vi "OCT_Run_sub.vi"(11 "saveing method":string(combo)="SaveQueueImages") -> (3 "Lumedica report":string)   [LabVIEW 2021]
uses:
  <vilib>/Instr/_visa.llb/Select Event Type.ctl
  <vilib>/Instr/_visa.llb/VISA Configure Serial Port (Instr).vi
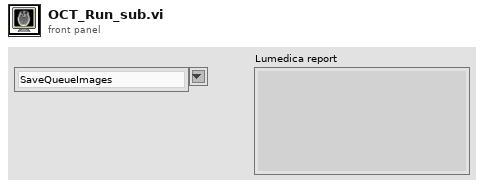
[diagram p1: front panel]
types:
  T1 = typedef "Select Event Type.ctl" = u32
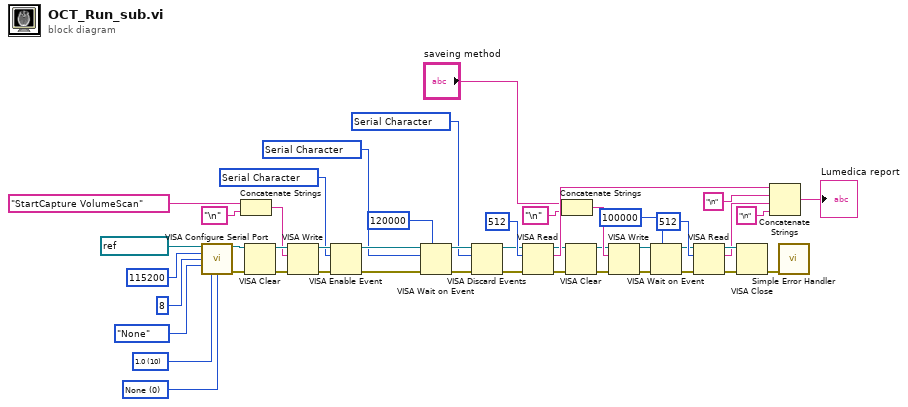
[diagram p0: block diagram]
diagram:
  w6 = T1 1073684533 items=["Service Request"=1073684491, "Trigger"=3221168138, "Clear"=1073684493, "VXI Signal"=1073684512, "VXI/VME Interrupt"=3221168161, "VXI/VME Sysfail"=1073684509, "VXI/VME Sysreset"=1073684510, "GPIB CIC"=1073684498, "GPIB Talk"=1073684499, "GPIB Listen"=1073684500, "PXI Interrupt"=1073684514, "Serial Break"=1073684515, "Serial TermChar"=1073684516, "Serial CTS"=1073684521, "Serial DSR"=1073684522, "Serial DCD"=1073684524, "Serial RI"=1073684526, "Serial Character"=1073684533, "USB Interrupt"=1073684535, "All Enabled"=1073709055] ("Event Type")
  w12 = T1 1073684533 items=["Service Request"=1073684491, "Trigger"=3221168138, "Clear"=1073684493, "VXI Signal"=1073684512, "VXI/VME Interrupt"=3221168161, "VXI/VME Sysfail"=1073684509, "VXI/VME Sysreset"=1073684510, "GPIB CIC"=1073684498, "GPIB Talk"=1073684499, "GPIB Listen"=1073684500, "PXI Interrupt"=1073684514, "Serial Break"=1073684515, "Serial TermChar"=1073684516, "Serial CTS"=1073684521, "Serial DSR"=1073684522, "Serial DCD"=1073684524, "Serial RI"=1073684526, "Serial Character"=1073684533, "USB Interrupt"=1073684535, "All Enabled"=1073709055] ("Event Type")
  w13 = T1 1073684533 items=["Service Request"=1073684491, "Trigger"=3221168138, "Clear"=1073684493, "VXI Signal"=1073684512, "VXI/VME Interrupt"=3221168161, "VXI/VME Sysfail"=1073684509, "VXI/VME Sysreset"=1073684510, "GPIB CIC"=1073684498, "GPIB Talk"=1073684499, "GPIB Listen"=1073684500, "PXI Interrupt"=1073684514, "Serial Break"=1073684515, "Serial TermChar"=1073684516, "Serial CTS"=1073684521, "Serial DSR"=1073684522, "Serial DCD"=1073684524, "Serial RI"=1073684526, "Serial Character"=1073684533, "USB Interrupt"=1073684535, "All Enabled"=1073709055] ("Event Type")
  w42 = u16 10 items=["1.0"=10, "1.5"=15, "2.0"=20] ("stop bits (10: 1 bit)")
  w41 = u16 0 items=["None", "XON/XOFF", "RTS/CTS", "XON/XOFF & RTS/CTS", "DTR/DSR", "XON/XOFF & DTR/DSR"] ("flow control (0:none)")
  n1 = call-poly "VISA Configure Serial Port"("VISA resource name"=refnum<visa-resource-name> "COM22", "baud rate (9600)"=u32 115200, "data bits (8)"=u16 8, "parity (0:none)"=enum16{"None", "Odd", "Even", "Mark", "Space"}."None", "stop bits (10: 1 bit)"=w42, "flow control (0:none)"=w41) -> ("VISA resource name out"=w40:refnum<visa-resource-name>, "error out"=w39:errorcluster)  [unwired: 4 in, 4 out]
  n2 = Concatenate Strings("StartCapture VolumeScan" ("write buffer"), "\n" ("write buffer")) -> (w34:string)
  n3 = VISA Clear(VISA resource name=w40, error in (no error)=w39) -> (VISA resource name out=w38:refnum<visa-resource-name>, error out=w37:errorcluster)
  n4 = VISA Write(VISA resource name=w38, write buffer=w34, error in (no error)=w37) -> (VISA resource name out=w17:refnum<visa-resource-name>, error out=w16:errorcluster)  [unwired: 1 out]
  n5 = VISA Enable Event(8:w16, 10:w13, 11:w17) -> (0:w14:errorcluster, 3:w15:refnum<visa-resource-name>)  [unwired: 1 in]
  n6 = VISA Wait on Event(7:u32 120000 ("timeout (0)"), 8:w14, 10:w12, 11:w15) -> (0:w9:errorcluster, 3:w10:refnum<visa-resource-name>)  [unwired: 1 in, 2 out]
  n7 = VISA Discard Events(8:w9, 10:w6, 11:w10) -> (0:w7:errorcluster, 3:w8:refnum<visa-resource-name>)  [unwired: 1 in]
  n8 = VISA Read(VISA resource name=w8, byte count=u32 512, error in (no error)=w7) -> (VISA resource name out=w28:refnum<visa-resource-name>, read buffer=w47:string, error out=w27:errorcluster)  [unwired: 1 out]
  n9 = Concatenate Strings("saveing method", "\n" ("write buffer")) -> (w32:string)
  n10 = VISA Clear(VISA resource name=w28, error in (no error)=w27) -> (VISA resource name out=w30:refnum<visa-resource-name>, error out=w33:errorcluster)
  n11 = VISA Write(VISA resource name=w30, write buffer=w32, error in (no error)=w33) -> (VISA resource name out=w5:refnum<visa-resource-name>, error out=w4:errorcluster)  [unwired: 1 out]
  n12 = VISA Wait on Event(7:u32 100000 ("timeout (0)"), 8:w4, 11:w5) -> (0:w2:errorcluster, 3:w3:refnum<visa-resource-name>)  [unwired: 2 in, 2 out]
  n13 = VISA Read(VISA resource name=w3, byte count=u32 512, error in (no error)=w2) -> (VISA resource name out=w22:refnum<visa-resource-name>, read buffer=w20:string, error out=w21:errorcluster)  [unwired: 1 out]
  n14 = VISA Close(VISA resource name=w22, error in (no error)=w21) -> (error out=w25:errorcluster)
  n15 = Concatenate Strings(w47, "\n" ("write buffer"), w20, "\n" ("write buffer")) -> (→"Lumedica report":string)
  n16 = call <vilib>:"Simple Error Handler.vi"("error in (no error)"=w25) -> ()  [unwired: 1 in, 8 out]
